vi "Exemple_Metrics_Matthews_Corrcoef.vi"() -> ()   [LabVIEW 2020]
uses:
  Objet/3 - Model selection and evaluation/3.3 - Metrics and scoring/matthews_corrcoef/Matthews_Corrcoef.vi
panel:
  out "Score":string
  out "error out":errorcluster caption="sortie d'erreur"
  in  "matthews_corrcoef":cluster{"sample_weight":dbl[]}
  in  "error in (no error)":errorcluster caption="entrée d'erreur (pas d'erreur)"
  in  "y_pred":string[][](array[string])=[["1"], ["-1"], ["1"], ["1"]]
  in  "y_true":string[][](array[string])=[["1"], ["1"], ["1"], ["-1"]]
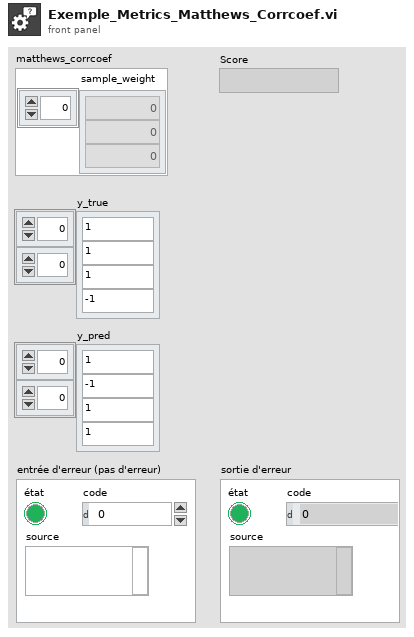
[diagram p1: front panel]
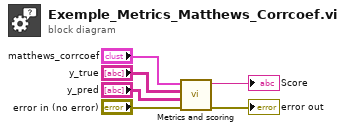
[diagram p0: block diagram]
diagram:
  n1 = call-poly "Metrics and scoring.vi"("error in (no error)"="error in (no error)", "y_pred"="y_pred", "y_true"="y_true", "matthews_corrcoef"="matthews_corrcoef") -> ("error out"=→"error out":errorcluster, "Score"=→"Score":string)  [unwired: 6 in]
